vi "ocv.vi"(0 "IP adress":string="192.109.209.229", 1 "stop":bool, 2 "Channel":u8(ring) items=["1", "2", "3", "4", "5", "6", "7", "8", "9", "10", "11", "12", "13", "14", "15", "16"], 3 "OCV Parameters":T1={"Rest_time_T"=1.0, "Record_every_dE"=0.01, "Record_every_dT"=0.01, "E_Range"=3, "em"=1, "ce"=0, "tb"=2e-05} {"tb" min=2e-05 max=1 format="%^_3e"; "ce" items=["Standard", "CE to ground"]; "E_Range" items=["±2.5V", "±5V", "±10V", "Auto"]; "Record_every_dT" min=0 format="%.2e"; "Record_every_dE" min=0 max=100 format="%.4f"; "Rest_time_T" min=0 format="%.2f"}, 4 "Exit":bool, 5 "Start":bool, 6 "Draw":enum16{"Ewe(t)", "Ece(t)"}(ring)) -> (7 "XY Graph":cluster{"Data 100":dbl[], "Data 100":dbl[]}(graph), 8 "Number of points":i32)   [LabVIEW 2012]
doc: "The Open Circuit Voltage technique consists of a period during which no potantial or current is applied to the working electrode.\nThis VI contain others sub VIs.\nIn general,in this VI, the first thing to do is to start by establishing the connection with the instrument defined by its IP adress, then load the firmware in the channel selected, get the information on the plugged channels, load protocol on a channel, start/stop the protocol, retreive data and draw the graph."
panel:
  in  "Update":bool caption="Start"
  out "Exit 2":bool
  out "Data 100":dbl[][](array[numeric]) format="%.2f"
  # "Instructions:\nBefore running the VI you must type a valid IP adress that corresponds to the instrument.Then press the Run button to execute this VI.\nWhile this VI is running, choose the available channel, enter the OCV parameters or keep the default values, then press the start button to begin the experience. \nThe potential response as a function of the time (Ewe(t), Ece(t)) will be drawn."
  # "Rest for time tr( s)"
  # "Record every dEr (V)"
  # "And at least every dtr (s)"
  # "E range"
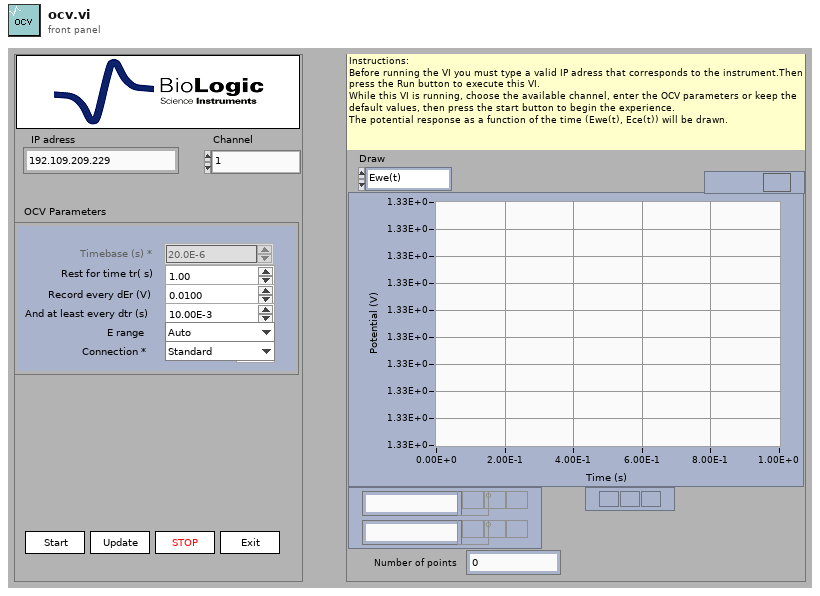
[diagram p1: front panel]
types:
  T1 = cluster{"Rest_time_T":sgl, "Record_every_dE":sgl, "Record_every_dT":sgl, "E_Range":u16, "em":u16, "ce":u16, "tb":sgl}
  T2 = cluster{"Label":string, "type":i32, "valeur":u32, "index":i32}[]
  T3 = cluster{"IRQskipped":i32, "NbRaws":i32, "NbCols":i32, "Technique Index":i32, "TechniqueID":i32, "PrcessIndex":i32, "loop":i32, "StartTime":dbl, "MuxPad":i32}
  T4 = cluster{"State":i32, "MemFilled":i32, "TimeBase":sgl, " Ewe":sgl, " EweRangeMin":sgl, " EweRangeMax":sgl, "Ece":sgl, "EceRangeMin":sgl, "EceRangeMax":sgl, "Eoverflow":i32, "I":sgl, "IRange":i32, "Ioverflow":i32, "ElapsedTime":sgl, "Freq":sgl, "Rcomp":sgl, "Saturation":sgl, "OptErr":i32, "OptPos":i32}
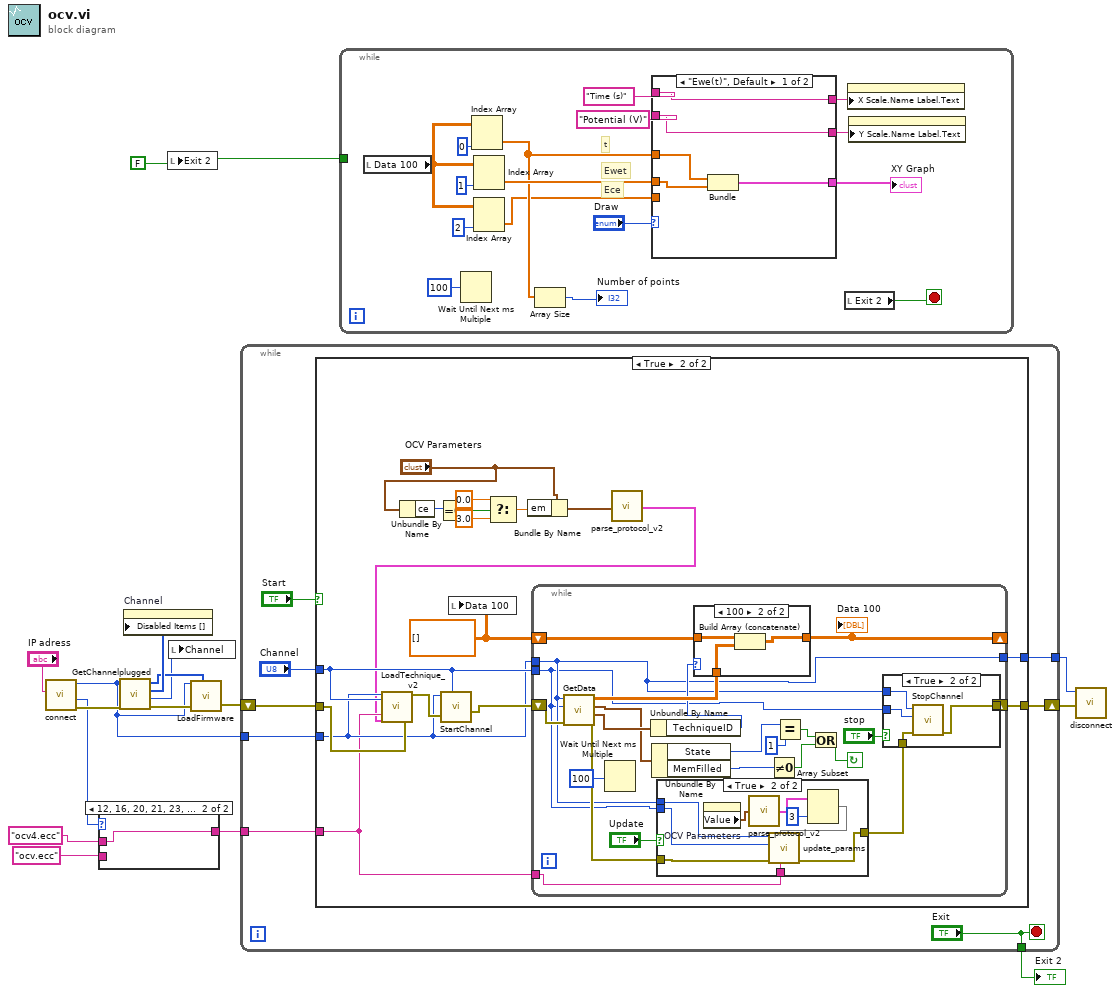
[diagram p0: block diagram]
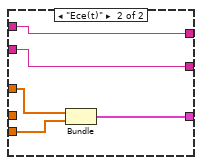
[diagram p3: hidden frame]
diagram:
  w15 = FALSE ("Exit 2")
  n1 = call "connect.vi"("IP"="IP adress") -> ("error out"=w13:errorcluster, "Device Code"=w2:i32, "ID"=w6:i32)  [unwired: 7 in, 1 out]
  n2 = case shown="12, 16, 20, 21, 23, 27" w2 {
    tunnel: "ocv.ecc" ("FName") -> [w17 _]
    tunnel: [w17 w18] -> w1
    tunnel: "ocv4.ecc" ("FName") -> [_ w18]
    frame Default {
    }
    frame 12, 16, 20, 21, 23, 27 {
    }
  }
  n3 = call "GetChannelplugged.vi"("error in (no error)"=w13, "ID"=w6) -> ("error out"=w10:errorcluster, "First channel"=w8:i32, "Disabled channels"=w12:i32[], "Plugged channels"=w11:i32[])  [unwired: 6 in]
  n4 = property on="Channel" class="Ring (strict)"("Disabled Items []"=w12) -> ()  [unwired: 2 in, 2 out]
  n5 = local write "Exit 2"(w15) -> ()
  n6 = local write "Channel"(w8) -> ()
  n7 = call "LoadFirmware.vi"("error in (no error)"=w10, "Channels"=w11, "ID"=w6) -> ("error out"=w7:errorcluster)  [unwired: 7 in, 1 out]
  n8 = while {
    shift-right: [w25] -> w14
    shift-left: w7 -> [w19]
    tunnel: ["Exit"] -> w16
    tunnel: w6 -> [w23]
    tunnel: [w22] -> w5
    tunnel: w1 -> [w20]
    stop <- "Exit" stop-if-true
    n9 = case shown="True" "Start" {
      tunnel: "Channel" -> [_ w42]
      tunnel: [w28 w43] -> w25
      tunnel: w19 -> [w28 w41]
      tunnel: w23 -> [w27 w39]
      tunnel: [w27 w38] -> w22
      tunnel: w20 -> [_ w31]
      frame False {
      }
      frame True {
        w40 = dbl[][] []
        n10 = Unbundle By Name("OCV Parameters") -> ("ce"=w33:u16)
        n11 = Equal To 0?(x=w33) -> (x = 0?=w32:bool)
        n12 = local write "Data 100"(w40) -> ()
        n13 = Select(t=0.0, s=w32, f=3.0) -> (s? t:f=w36:dbl)
        n14 = Bundle By Name(cluster="OCV Parameters", "em"=w36) -> (w30:T1)
        n15 = call "parse_protocol_v2.vi"("Protocol Cluster"=w30) -> ("Params Values"=w29:T2)
        n16 = call "LoadTechnique_v2.vi"("ID"=w39, "Selected Channel"=w42, "FName"=w31, "Protocol Parameters"=w29, "error in (no error)"=w41) -> ("error out"=w45:errorcluster)  [unwired: 14 in]
        n17 = call "StartChannel.vi"("error in (no error)"=w45, "Channel"=w42, "ID"=w39) -> ("error out"=w44:errorcluster)  [unwired: 8 in]
        n18 = while {
          shift-right: [w61] -> w43
          shift-left: w44 -> [w64]
          shift-right: [w59] -> _
          shift-left: w40 -> [w58]
          tunnel: w42 -> [w47]
          tunnel: w39 -> [w48]
          tunnel: [w48] -> w38
          tunnel: w31 -> [w46]
          stop <- w62 continue-if-true
          n19 = call "GetData.vi"("error in (no error)"=w64, "Channel"=w47, "ID"=w48) -> ("error out"=w50:errorcluster, "Data information"=w55:T3, "Current values"=w52:T4, "Data"=w60:dbl[][])  [unwired: 5 in]
          n20 = Wait Until Next ms Multiple(millisecond multiple=u32 100) -> ()  [unwired: 1 out]
          n21 = Unbundle By Name(w55) -> ("TechniqueID"=w56:i32)
          n22 = Unbundle By Name(w52) -> ("State"=w54:i32, "MemFilled"=w53:i32)
          n23 = case shown="True" "Update" {
            tunnel: w50 -> [w68 w77]
            tunnel: [w68 w76] -> w49
            tunnel: w48 -> [_ w75]
            tunnel: w47 -> [_ w74]
            tunnel: w46 -> [_ w73]
            frame False {
            }
            frame True {
              n24 = property on="OCV Parameters" class="Clust (strict)"() -> ("Value"=w72:T1)  [unwired: 2 in, 2 out]
              n25 = call "parse_protocol_v2.vi"("Protocol Cluster"=w72) -> ("Params Values"=w71:T2)
              n26 = Array Subset(array=w71, length=3) -> (w69:T2)  [unwired: 1 in]
              n27 = call "update_params.vi"("EccFileName"=w73, "Params"=w69, "error in (no error)"=w77, "Channel"=w74, "ID"=w75) -> ("error out"=w76:errorcluster)  [unwired: 6 in]
            }
          }
          n28 = case shown="100" w56 {
            tunnel: w60 -> [_ w86]
            tunnel: [w83 w85] -> w59
            tunnel: w58 -> [w83 w84]
            frame 0, Default {
            }
            frame 100 {
              n29 = Build Array (concatenate)(w84, w86) -> (w85:dbl[][])
            }
          }
          "Data 100" <- w59
          n30 = Not Equal To 0?(x=w53) -> (x != 0?=w65:bool)
          n31 = Equal?(x=w54, y=1) -> (x = y?=w66:bool)
          n32 = Or(x=w66, y=w65) -> (x .or. y?=w62:bool)
          n33 = case shown="True" "stop" {
            tunnel: [w78 w82] -> w61
            tunnel: w49 -> [w78 w81]
            tunnel: w47 -> [_ w80]
            tunnel: w48 -> [_ w79]
            frame False {
            }
            frame True {
              n34 = call "StopChannel.vi"("error in (no error)"=w81, "Channel"=w80, "ID"=w79) -> ("error out"=w82:errorcluster)  [unwired: 8 in]
            }
          }
        }
      }
    }
  }
  "Exit 2" <- w16
  n35 = while {
    tunnel: w15 -> [_]
    stop <- w99 stop-if-true
    # "Ece"
    # "Ewet"
    # "t"
    n36 = local read "Data 100"() -> (w97:dbl[][])
    n37 = Wait Until Next ms Multiple(millisecond multiple=u32 100) -> ()  [unwired: 1 out]
    n38 = Index Array(array=w97, index (col)=0 ("Index")) -> (element=w90:dbl[])  [unwired: 1 in]
    n39 = Index Array(array=w97, index (col)=1 ("Index")) -> (element=w91:dbl[])  [unwired: 1 in]
    n40 = Index Array(array=w97, index (col)=2 ("indice désactivé (col)")) -> (element=w89:dbl[])  [unwired: 1 in]
    n41 = Array Size(array=w90) -> (size(s)=→"Number of points":i32)
    n42 = case shown="\"Ewe(t)\", Default" "Draw" {
      tunnel: "Time (s)" ("Y Scale.Name Label.Text") -> [w107 w112]
      tunnel: [w107 w112] -> w94
      tunnel: "Potential (V)" ("Y Scale.Name Label.Text") -> [w106 w111]
      tunnel: [w106 w111] -> w92
      tunnel: w90 -> [w105 w108]
      tunnel: w91 -> [w104 _]
      tunnel: w89 -> [_ w110]
      tunnel: [w103 w109] -> w87
      frame "Ewe(t)", Default {
        n43 = Bundle("Data 100"=w105, "Data 100"=w104) -> (w103:cluster{"Data 100":dbl[], "Data 100":dbl[]})  [unwired: 1 in]
      }
      frame "Ece(t)" {
        n44 = Bundle("Data 100"=w108, "Data 100"=w110) -> (w109:cluster{"Data 100":dbl[], "Data 100":dbl[]})  [unwired: 1 in]
      }
    }
    "XY Graph" <- w87
    n45 = local read "Exit 2"() -> (w99:bool)
    n46 = property on="XY Graph" class="XYGraph (strict)"("X Scale.Name Label.Text"=w94) -> ()  [unwired: 2 in, 2 out]
    n47 = property on="XY Graph" class="XYGraph (strict)"("Y Scale.Name Label.Text"=w92) -> ()  [unwired: 2 in, 2 out]
  }
  n48 = call "disconnect.vi"("error in (no error)"=w14, "ID"=w5) -> ()  [unwired: 9 in, 1 out]
